vi "协议-向设备设置服务器信息.vi"(8 "端口":u16, 9 "IP地址":string, 11 "服务器/上位机？":enum8{"服务器", "上位机"}(ring)) -> (3 "完整输出":string)   [LabVIEW 2013]
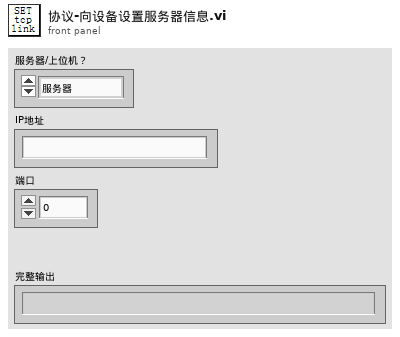
[diagram p1: front panel]
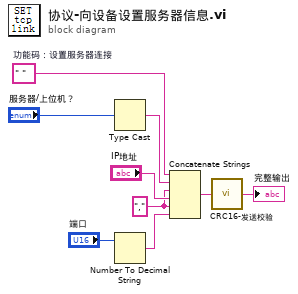
[diagram p0: block diagram]
diagram:
  w1 = ","
  w3 = " "  # 功能码：设置服务器连接
  n1 = Type Cast(x="服务器/上位机？") -> (*(type *) &x=w2:string)  [unwired: 1 in]
  n2 = Number To Decimal String(number="端口") -> (decimal integer string=w6:string)  [unwired: 1 in]
  n3 = Concatenate Strings(w3, w2, w1, "IP地址", w1, w6) -> (w5:string)
  n4 = call "CRC16-发送校验.vi"("净数据"=w5) -> ("完整输出"=→"完整输出":string)
